vi "Read dB Ref.vi"(8 "error in (no error)":errorcluster, 11 "Dynamic in":refnum<class "Dynamic.lvclass">) -> (0 "error out":errorcluster, 2 "dB Ref":dbl, 3 "Dynamic out":refnum<class "Dynamic.lvclass">)   [LabVIEW 2018, in "Measurement Channels.lvlib" / "Dynamic.lvclass"]
uses:
  Dynamic.lvclass
  Dynamic.lvclass/Dynamic.ctl
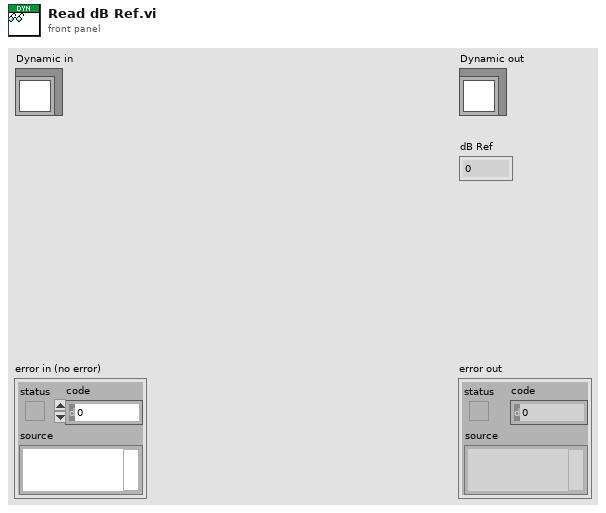
[diagram p1: front panel]
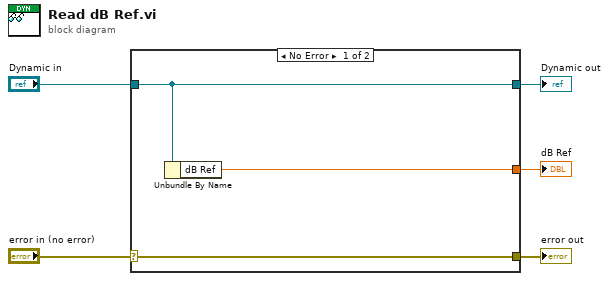
[diagram p0: block diagram]
diagram:
  n1 = case shown="No Error" "error in (no error)" {
    selector: "error in (no error)" -> [w8 w9]
    tunnel: [w8 w9] -> w4
    tunnel: [w7 w10] -> w2
    tunnel: "Dynamic in" -> [w7 w10]
    tunnel: [w6 _] -> w1
    frame No Error {
      n2 = Unbundle By Name(w7) -> ("dB Ref"=w6:dbl)
    }
    frame Error {
    }
  }
  "error out" <- w4
  "Dynamic out" <- w2
  "dB Ref" <- w1
